vi "Daemon.vi"(4 "Length":T1, 6 "Interrupts":T2, 8 "Port Type":enum8{"CMD", "TLM", "BOTH"}(ring), 9 "Port":u16, 10 "Target Queue":refnum<queue>, 11 "Connection":refnum<data-value>) -> ()   [LabVIEW 2018, in "TCPServer.lvlib"]
uses:
  TCPServer.lvlib
  TypeDefs/Connection.ctl
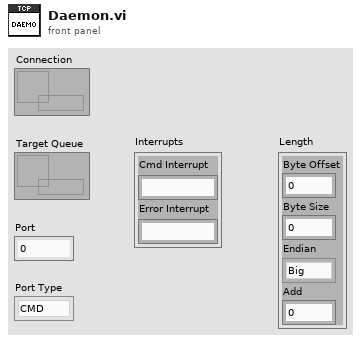
[diagram p1: front panel]
types:
  T1 = cluster{"Byte Offset":i32, "Byte Size":i32, "Endian":enum8{"Big", "Little"}, "Add":i32}
  T2 = cluster{"Cmd Interrupt":string, "Error Interrupt":string}
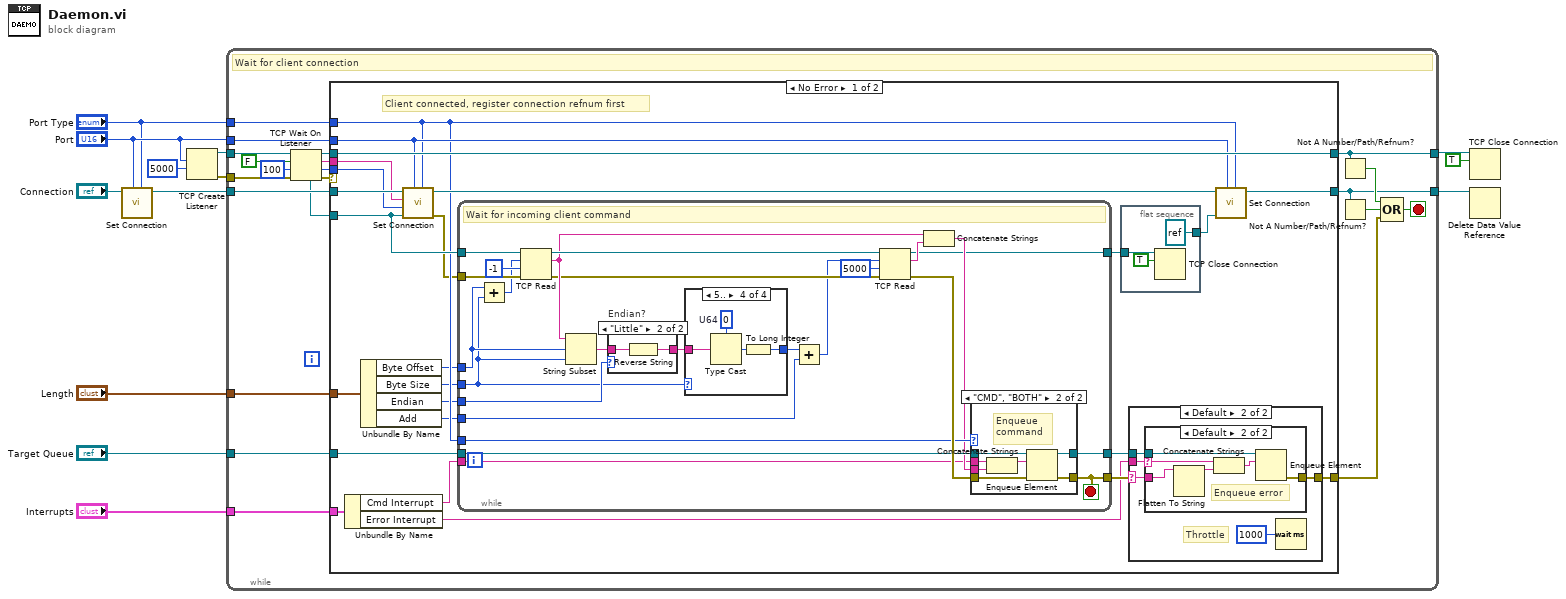
[diagram p0: block diagram]
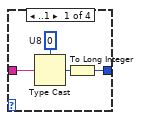
[diagram p2: hidden frame]
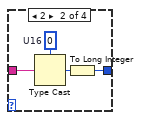
[diagram p3: hidden frame]
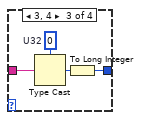
[diagram p4: hidden frame]
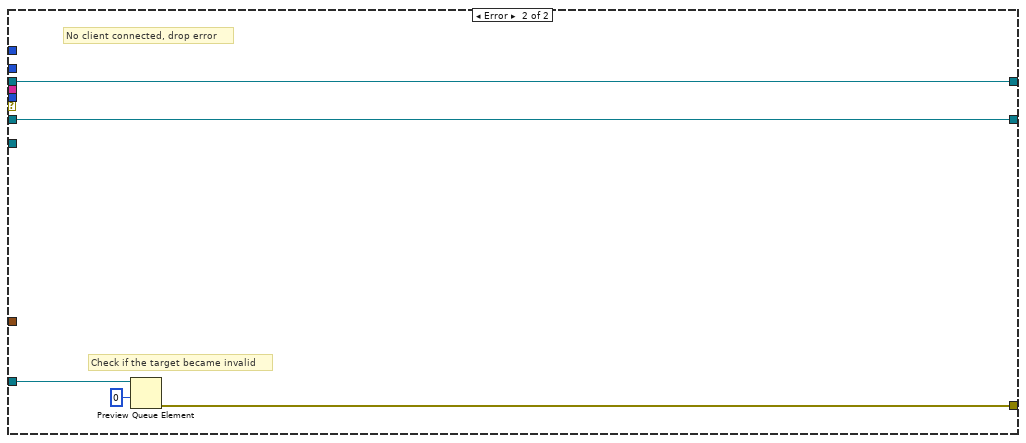
[diagram p9: hidden frame]
diagram:
  n1 = call "Set Connection.vi"("Server Port Type"="Port Type", "Server Port"="Port", "Connection in"="Connection") -> ("Connection out"=w5:refnum<data-value>)  [unwired: 7 in, 1 out]
  n2 = TCP Create Listener(9:5000 ("timeout ms (25000)"), 10:"Port") -> (0:w12:errorcluster, 3:w13:refnum<k5>)  [unwired: 3 in, 1 out]
  n3 = while {
    tunnel: w13 -> [w34]
    tunnel: w12 -> [w33]
    tunnel: w5 -> [w29]
    tunnel: "Port Type" -> [w27]
    tunnel: "Target Queue" -> [w26]
    tunnel: [w23] -> w10
    tunnel: [w17] -> w8
    tunnel: "Port" -> [w20]
    tunnel: "Length" -> [w15]
    tunnel: "Interrupts" -> [w14]
    stop <- w22 stop-if-true
    # "Wait for client connection"
    n4 = TCP Wait On Listener(8:w33, 9:100 ("timeout ms (wait forever: -1)"), 10:FALSE ("resolve remote address (T)"), 11:w34) -> (0:w30:errorcluster, 1:w18:u16, 2:w19:string, 3:w25:refnum<k5>, 4:w28:refnum<k5>)
    n5 = case shown="No Error" w30 {
      tunnel: w29 -> [w52 w130]
      tunnel: w28 -> [w51 _]
      tunnel: w27 -> [w45 _]
      tunnel: w26 -> [w58 w128]
      tunnel: [w47 w130] -> w17
      tunnel: w25 -> [w57 w129]
      tunnel: [w57 w129] -> w23
      tunnel: [w53 w126] -> w21
      tunnel: w20 -> [w46 _]
      tunnel: w19 -> [w49 _]
      tunnel: w18 -> [w50 _]
      tunnel: w15 -> [w42 _]
      tunnel: w14 -> [w37 _]
      frame No Error {
        # "Client connected, register connection refnum first"
        n6 = Unbundle By Name(w37) -> ("Cmd Interrupt"=w36:string, "Error Interrupt"=w35:string)
        n7 = Unbundle By Name(w42) -> ("Byte Offset"=w41:i32, "Byte Size"=w40:i32, "Endian"=w39:enum8{"Big", "Little"}, "Add"=w38:i32)
        n8 = call "Set Connection.vi"("Server Port Type"=w45, "Server Port"=w46, "Client"=w51, "Client Port"=w50, "Client IP"=w49, "Connection in"=w52) -> ("error out"=w44:errorcluster, "Connection out"=w48:refnum<data-value>)  [unwired: 4 in]
        n9 = while {
          tunnel: w44 -> [w85]
          tunnel: w51 -> [w84]
          tunnel: w58 -> [w79]
          tunnel: w45 -> [w78]
          tunnel: w36 -> [w76]
          tunnel: [w75] -> w54
          tunnel: [w74] -> w56
          tunnel: [w73] -> w55
          tunnel: w41 -> [w70]
          tunnel: w40 -> [w62]
          tunnel: w38 -> [w67]
          tunnel: w39 -> [w63]
          stop <- w75 stop-if-true
          # "Wait for incoming client command"
          n10 = Add(x=w70, y=w62) -> (x+y=w72:i32)
          n11 = TCP Read(connection ID=w84, bytes to read=w72, error in (no error)=w85, 9:-1 ("timeout ms (25000)")) -> (connection ID out=w86:refnum<k5>, data out=w71:string, error out=w66:errorcluster)  [unwired: 1 in]
          n12 = String Subset(string=w71, offset (0)=w70, length (rest)=w62) -> (substring=w69:string)
          n13 = case "Endian?" shown="\"Little\"" w63 {
            tunnel: w69 -> [w103 w105]
            tunnel: [w103 w104] -> w64
            frame "Big" {
            }
            frame "Little" {
              n14 = Reverse String(1:w105) -> (0:w104:string)
            }
          }
          n15 = case shown="5.." w62 {
            tunnel: [w88 w92 w96 w100] -> w68
            tunnel: w64 -> [w87 w91 w95 w99]
            frame ..1 {
              w90 = u8 0  # U8
              n16 = Type Cast(type=w90, x=w87) -> (*(type *) &x=w89:u8)
              n17 = To Long Integer(number=w89) -> (32bit integer=w88:i32)
            }
            frame 2 {
              w94 = u16 0  # U16
              n18 = Type Cast(type=w94, x=w91) -> (*(type *) &x=w93:u16)
              n19 = To Long Integer(number=w93) -> (32bit integer=w92:i32)
            }
            frame 3, 4 {
              w98 = u32 0  # U32
              n20 = Type Cast(type=w98, x=w95) -> (*(type *) &x=w97:u32)
              n21 = To Long Integer(number=w97) -> (32bit integer=w96:i32)
            }
            frame 5.. {
              w102 = u64 0  # U64
              n22 = Type Cast(type=w102, x=w99) -> (*(type *) &x=w101:u64)
              n23 = To Long Integer(number=w101) -> (32bit integer=w100:i32)
            }
          }
          n24 = Add(x=w68, y=w67) -> (x+y=w65:i32)
          n25 = TCP Read(connection ID=w86, bytes to read=w65, error in (no error)=w66, 9:5000 ("timeout ms (25000)")) -> (connection ID out=w74:refnum<k5>, data out=w81:string, error out=w80:errorcluster)  [unwired: 1 in]
          n26 = Concatenate Strings(w71, w81) -> (w77:string)
          n27 = case shown="\"CMD\", \"BOTH\"" w78 {
            tunnel: w80 -> [w107 w114]
            tunnel: w79 -> [w106 w113]
            tunnel: w77 -> [_ w112]
            tunnel: w76 -> [_ w111]
            tunnel: [w107 w109] -> w75
            tunnel: [w106 w108] -> w73
            frame "TLM" {
              # "Ignore\ntelemetry"
            }
            frame "CMD", "BOTH" {
              # "Enqueue\ncommand"
              n28 = Concatenate Strings(w111, w112) -> (w110:string)
              n29 = Enqueue Element(queue=w113, element=w110, error in (no error)=w114) -> (queue out=w108:refnum<queue>, error out=w109:errorcluster)  [unwired: 1 in, 1 out]
            }
          }
        }
        n30 = flat-sequence {
          tunnel: w56 -> [w61]
          tunnel: [refnum<k5> refnum ("Client")] -> w43
          frame #0 {
            n31 = TCP Close Connection(connection ID=w61, abort (F)=TRUE) -> ()  [unwired: 1 in, 2 out]
          }
        }
        n32 = case shown="Default" w54 {
          selector: w54 -> [_ w118]
          tunnel: w55 -> [_ w119]
          tunnel: w35 -> [_ w117]
          tunnel: [_ w116] -> w53
          frame "1", "66", "No Error" {
            # "1: Invalid queue\n66: Conection closed"
          }
          frame Default {
            # "Throttle"
            n33 = case shown="Default" w117 {
              selector: w117 -> [_ w122]
              tunnel: w119 -> [_ w124]
              tunnel: w118 -> [_ w123]
              tunnel: [_ w120] -> w116
              frame "" {
              }
              frame Default {
                # "Enqueue error"
                n34 = Flatten To String(anything=w123) -> (data string=w121:string)  [unwired: 3 in, 2 out]
                n35 = Concatenate Strings(w122, w121) -> (w125:string)
                n36 = Enqueue Element(queue=w124, element=w125) -> (error out=w120:errorcluster)  [unwired: 2 in, 2 out]
              }
            }
            n37 = Wait (ms)(milliseconds to wait=u32 1000) -> ()  [unwired: 1 out]
          }
        }
        n38 = call "Set Connection.vi"("Server Port Type"=w45, "Server Port"=w46, "Client"=w43, "Connection in"=w48) -> ("Connection out"=w47:refnum<data-value>)  [unwired: 6 in, 1 out]
      }
      frame Error {
        # "Check if the target became invalid"
        # "No client connected, drop error"
        n39 = Preview Queue Element(queue=w128, timeout in ms (-1)=0) -> (error out=w126:errorcluster)  [unwired: 1 in, 3 out]
      }
    }
    n40 = Not A Number/Path/Refnum?(number/path/refnum=w23) -> (NaN/Path/Refnum?=w24:bool)
    n41 = Not A Number/Path/Refnum?(number/path/refnum=w17) -> (NaN/Path/Refnum?=w16:bool)
    n42 = Compound Arithmetic op=OR(w24, w16, w21) -> (w22:bool)
  }
  n43 = TCP Close Connection(connection ID=w10, abort (F)=TRUE) -> ()  [unwired: 1 in, 2 out]
  n44 = Delete Data Value Reference(data value reference=w8) -> ()  [unwired: 1 in, 2 out]
